vi "takepressure.vi"() -> ()   [LabVIEW 2011]
uses:
  <vilib>/Utility/file.llb/Write To Spreadsheet File (DBL).vi
panel:
  out "Shot Number":i32
  in  "Tree":string="machine"
  in  "Time Node Path":string="pressure:p2_ion_gauge:time"
  in  "Voltage Node Path":string="pressure:p2_ion_gauge:signal"
  in  "Save Data File":path=path "C:/Documents and Settings/Helimak/My Documents/carterdodd/IonGauge/data.txt"
  out "Voltage Output":dynamicdata(graph)
  in  "Sample Rate":dbl=10.0
  in  "Sampling Time":dbl=60.0
  in  "Start Event":string="Shot_Init"
  out "Connect status":i32
  in  "Host":string="shanghai.ph.utexas.edu"
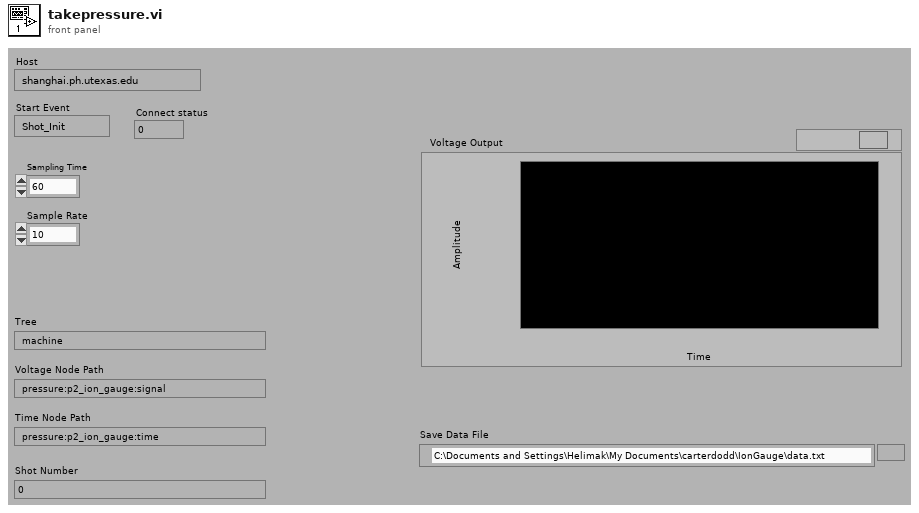
[diagram p1: front panel]
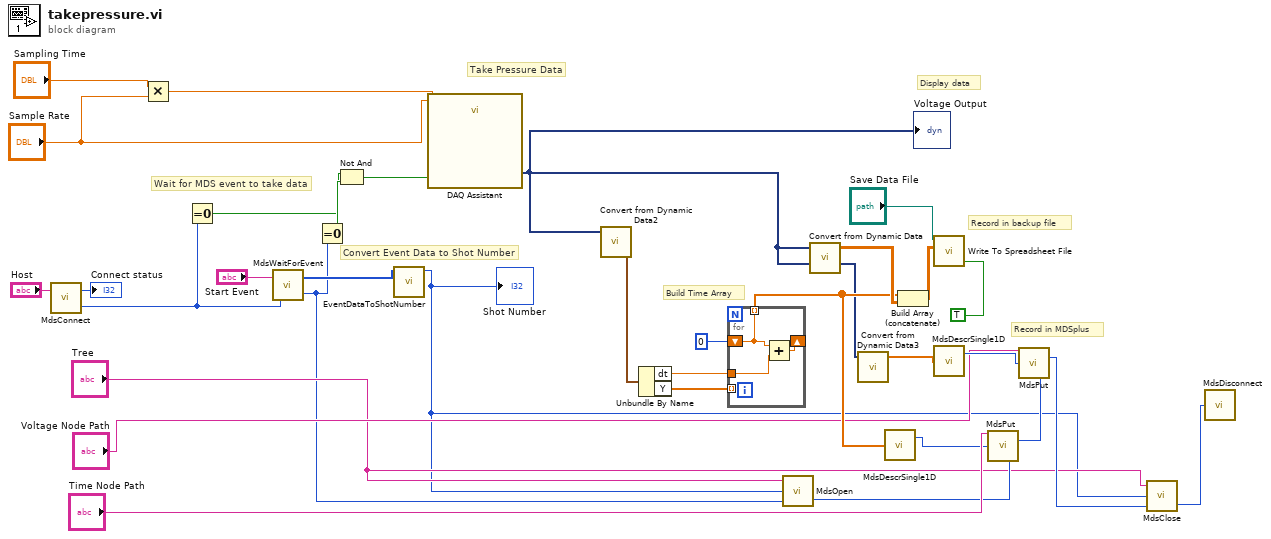
[diagram p0: block diagram]
diagram:
  # "Display data"
  # "Wait for MDS event to take data"
  # "Build Time Array"
  # "Record in MDSplus"
  # "Record in backup file"
  # "Take Pressure Data"
  # "Convert Event Data to Shot Number"
  n1 = call "MdsConnect.vi"("Host"="Host") -> ("FlowControlOut"=w30:i32, "Status"=→"Connect status":i32)  [unwired: 1 in]
  n2 = Multiply(x="Sampling Time", y="Sample Rate") -> (x*y=w24:dbl)
  n3 = Equal To 0?(x=w30) -> (x = 0?=w28:bool)
  n4 = call "MdsWaitForEvent.vi"("FlowControlIn"=w30, "Event"="Start Event") -> ("FlowControlOut"=w1:i32, "EventData"=w3:u8[])
  n5 = Equal To 0?(x=w1) -> (x = 0?=w29:bool)
  n6 = Not And(1:w29, 2:w28) -> (0:w27:bool)
  n7 = call "EventDataToShotNumber.vi"("EventDataIn"=w3) -> ("ShotNumberOut"=w2:i32)  [unwired: 10 in]
  "Shot Number" <- w2
  n8 = call "DAQ Assistant"("rate"="Sample Rate", "number of samples"=w24, "stop (T)"=w27) -> ("data"=w12:dynamicdata)  [unwired: 14 in, 2 out]
  "Voltage Output" <- w12
  n9 = call "Convert from Dynamic Data2"("Dynamic Data Type"=w12) -> ("Waveform"=w20:waveform(dbl))  [unwired: 3 in]
  n10 = Unbundle By Name(w20) -> ("dt"=w19:dbl, "Y"=w18:dbl[])
  n11 = for {
    shift-right: [w35] -> _
    shift-left: 0 -> [w34]
    tunnel: w19 -> [w36]
    tunnel: [w34] -> w15 mode=indexing
    tunnel: w18 -> [_] mode=indexing
    n12 = Add(x=w34, y=w36) -> (x+y=w35:dbl)
  }
  n13 = call "MdsOpen.vi"("FlowControlIn"=w1, "Shot"=w2, "Tree"="Tree") -> ("FlowControlOut"=w7:i32)  [unwired: 1 out]
  n14 = call "Convert from Dynamic Data"("Dynamic Data Type"=w12) -> ("Array"=w16:dbl[][])  [unwired: 3 in]
  n15 = call "Convert from Dynamic Data3"("Dynamic Data Type"=w12) -> ("Array"=w11:dbl[])  [unwired: 3 in]
  n16 = call "MdsDescrSingle1D.vi"("valueIn"=w15) -> ("DescrId"=w13:i32)  [unwired: 1 out]
  n17 = Build Array (concatenate)(w15, w16) -> (w17:dbl[][])
  n18 = call-poly <vilib>:"Write To Spreadsheet File.vi"("transpose? (no:F)"=TRUE, "2D data"=w17, "file path (dialog if empty)"="Save Data File") -> ()  [unwired: 5 in, 1 out]
  n19 = call "MdsDescrSingle1D.vi"("valueIn"=w11) -> ("DescrId"=w10:i32)  [unwired: 1 out]
  n20 = call "MdsPut.vi"("NodePath"="Time Node Path", "Descr1"=w13, "FlowControlIn"=w7) -> ("FlowControlOut"=w8:i32)  [unwired: 11 in, 1 out]
  n21 = call "MdsPut.vi"("NodePath"="Voltage Node Path", "Descr1"=w10, "FlowControlIn"=w8) -> ("FlowControlOut"=w6:i32)  [unwired: 11 in, 1 out]
  n22 = call "MdsClose.vi"("FlowControlIn"=w6, "Shot"=w2, "Tree"="Tree") -> ("FlowControlOut"=w4:i32)  [unwired: 1 out]
  n23 = call "MdsDisconnect.vi"("FlowControlIn"=w4) -> ()  [unwired: 1 out]
